vi "0MAIN.vi"() -> ()   [LabVIEW 2014]
uses:
  <vilib>/Instr/_visa.llb/VISA Configure Serial Port (Instr).vi
  <vilib>/Instr/_visa.llb/VISA Open Access Mode.ctl
panel:
  out "Пересчитано":bool=TRUE
  out "Метка получена 2":bool
  out "Время старта":string
  out "Ошибка файла":errorcluster
  out "Метка получена":bool
  out "Файл данных":refnum<file>
  out "Файл журнала":refnum<file>
  out "Номер метки":bool=TRUE
  out "error out 2":errorcluster
  in  "Управление":enum32{"Отладка", "График", "Настройки"}(tab)
  in  "Пересчитать в частоты":bool
  in  "Частота метки 2":bool
  in  "Записать данные":bool
  in  "Очистка буфера":bool
  in  "Чтение данных":bool
  in  "Установить":string
  in  "Отправка":bool
  out "Данные с МК":string
  out "Развертка X (В/ГГц)":dbl[](array[numeric])
  out "Сигнал Y (В)":dbl[](array[numeric])
  out "Метки (В, ГГц)":dbl[][](array[numeric])
  in  "Частота метки":bool
  in  "Выход":bool
  in  "Расчет графика":bool
  out "Индикатор КСВН":T1(graph)
  in  "Путь к файлу данных":path
  in  "Путь к логу":path
  in  "Логирование":bool
  out "Ошибка":T2
  in  "Порт":refnum<visa-resource-name>
  in  "Скорость передачи (9600)":u32=9600
  in  "Символ окончания (\\n)":u8=10 format="%.0x"
  in  "Режим доступа":T3 items=["VISA Defaults"=0, "Exclusive Lock"=1, "Load Configured Settings"=4]
  in  "Бит данных (8)":u8=8 format="%.0x"
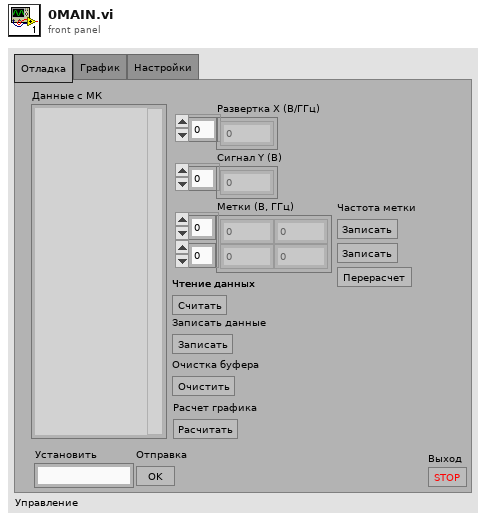
[diagram p1: front panel]
types:
  T1 = cluster{"Развертка X (В)":dbl[], "Сигнал Y (В)":dbl[]}
  T2 = cluster{"Статус":bool, "Код":i32, "Источник":string}
  T3 = typedef "VISA Open Access Mode.ctl" = u32
  T4 = enum16{"open", "replace", "create", "open or create", "replace or create", "replace or create with confirmation"}
  T5 = typedef "NI_Matrix.lvlib/RealMatrix.ctl" = dbl[][]
  T6 = cluster{"Развертка X (В/ГГц)":dbl[], "Сигнал Y (В)":dbl[]}
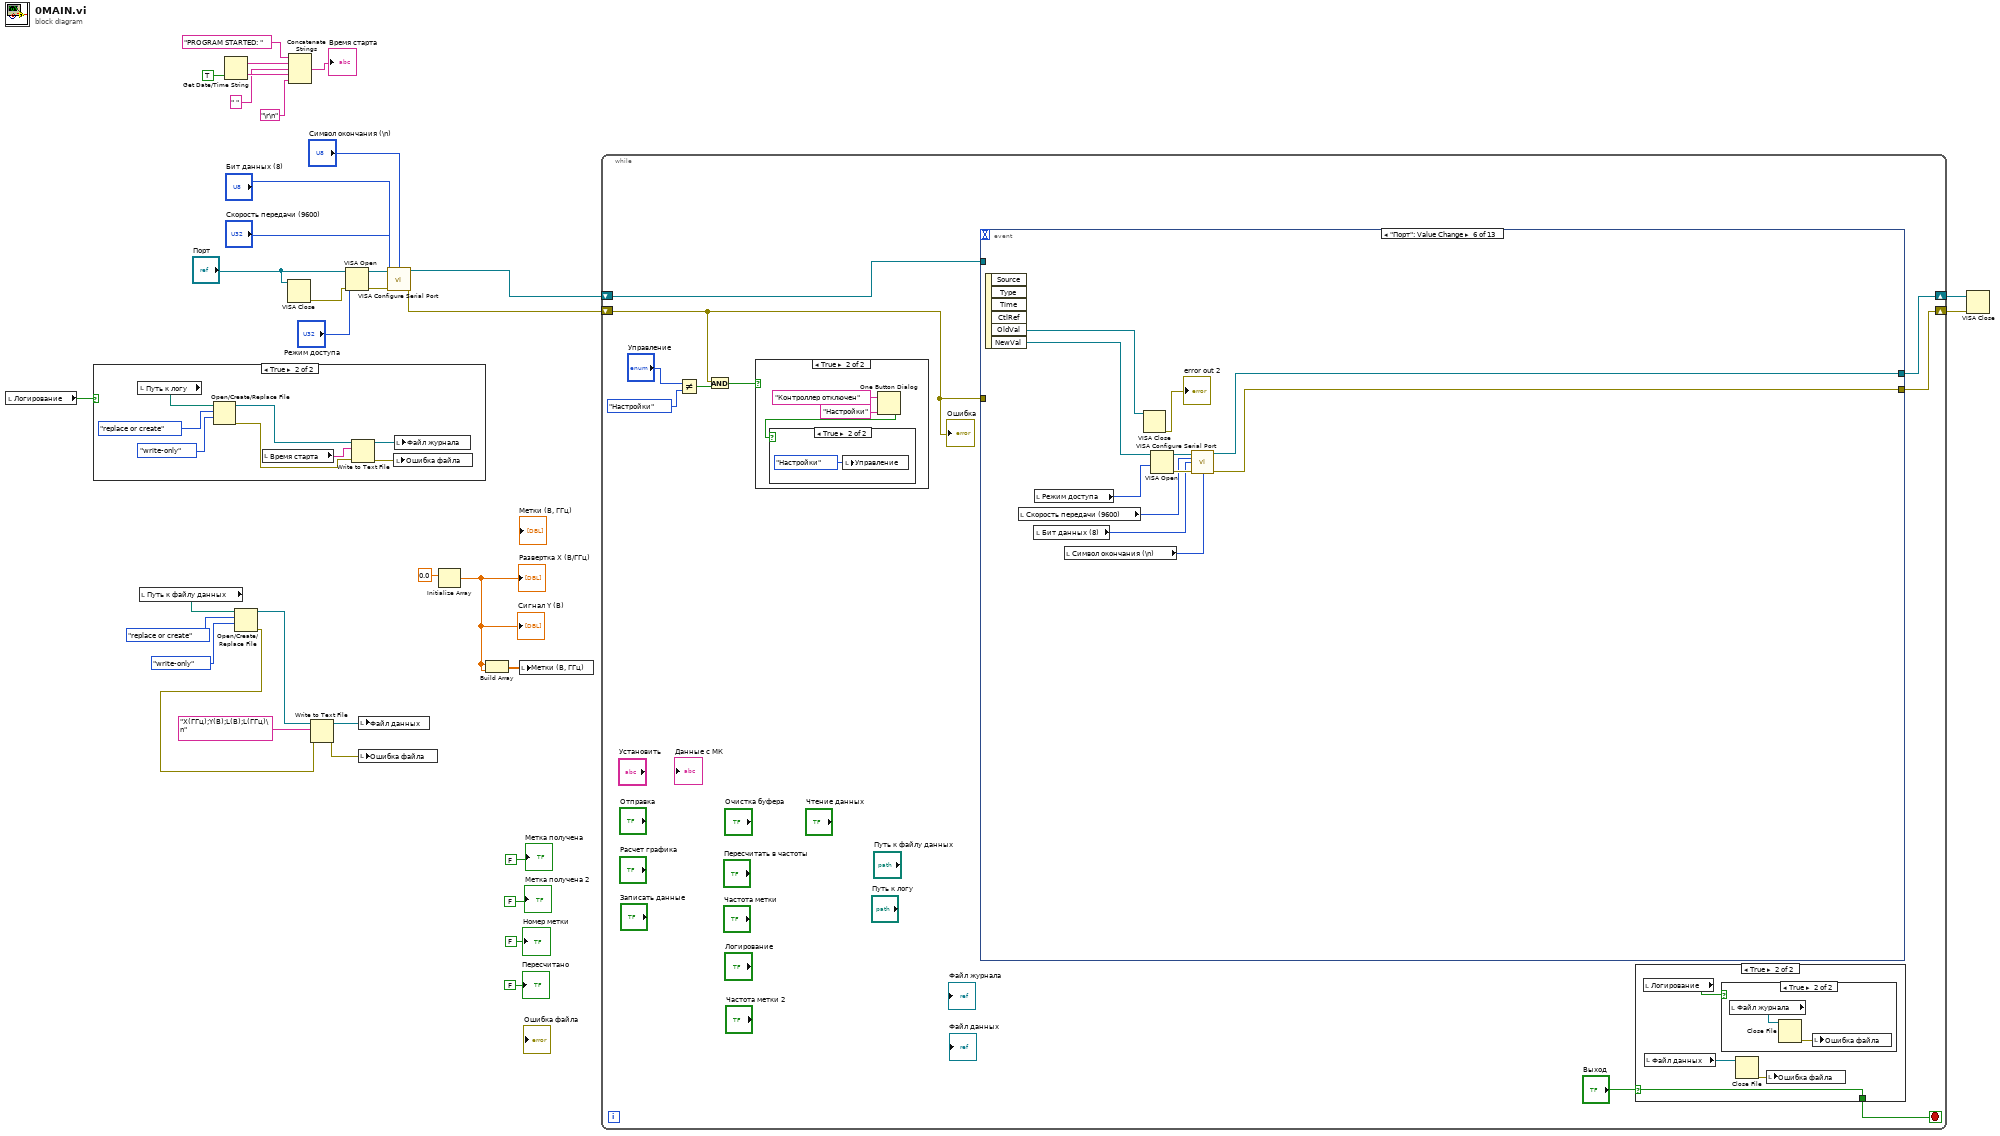
[diagram p0: block diagram]
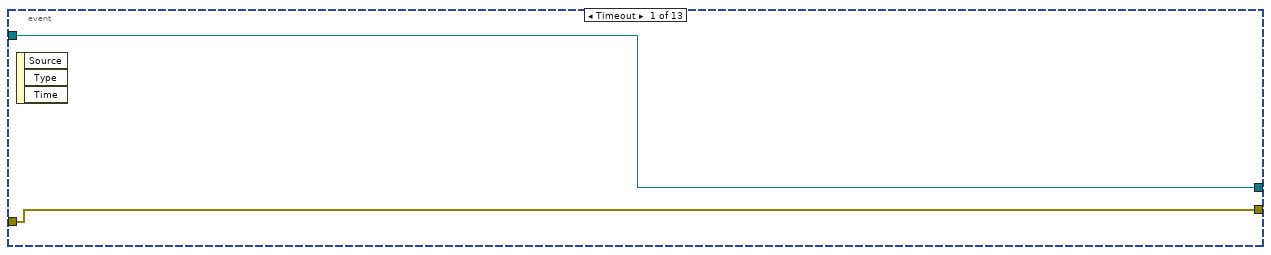
[diagram p7: hidden frame]
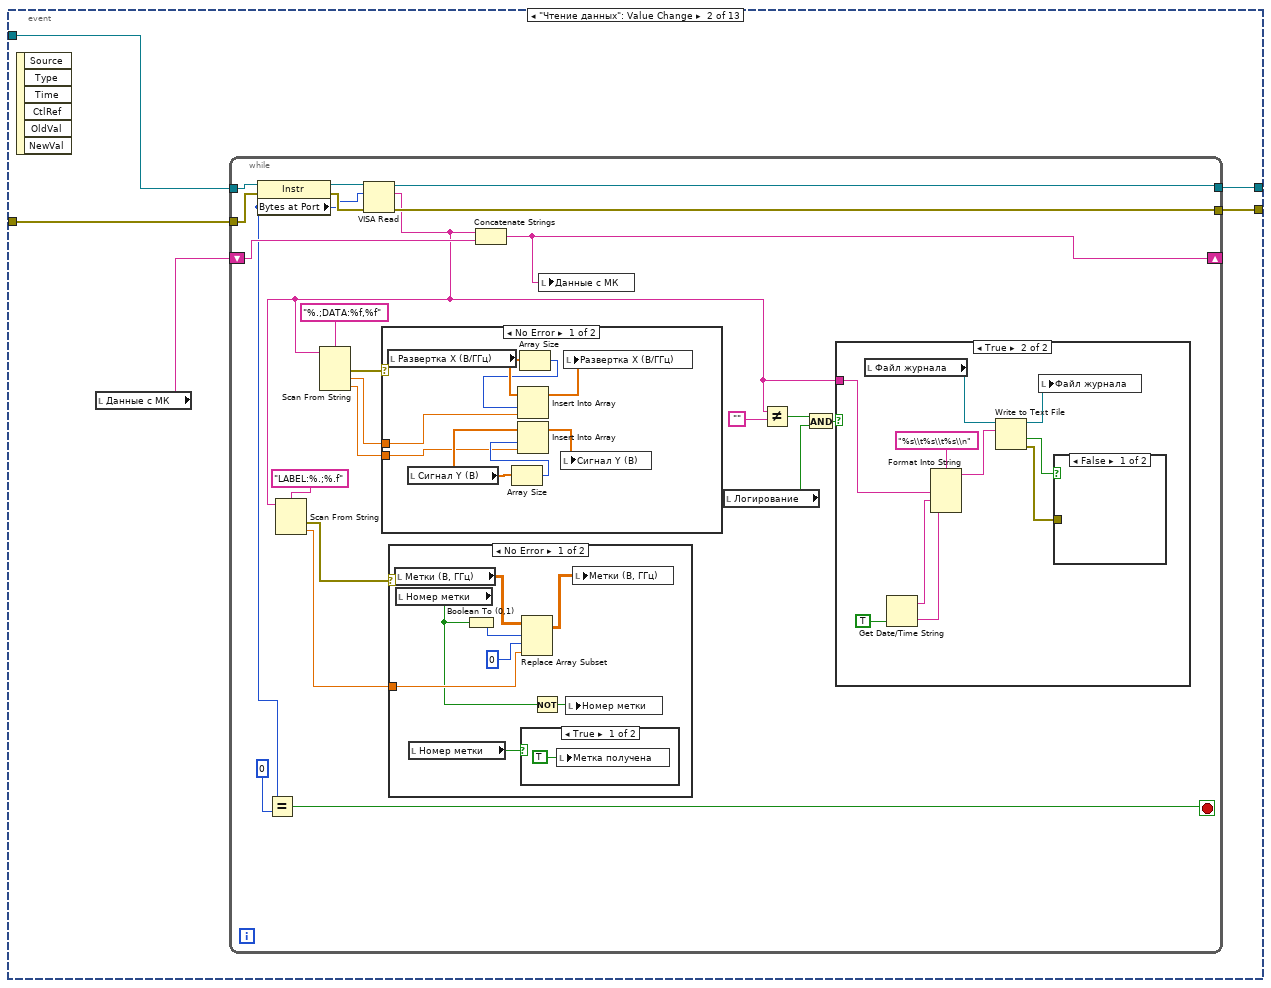
[diagram p8: hidden frame]
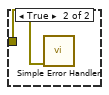
[diagram p10: hidden frame]
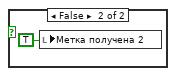
[diagram p11: hidden frame]
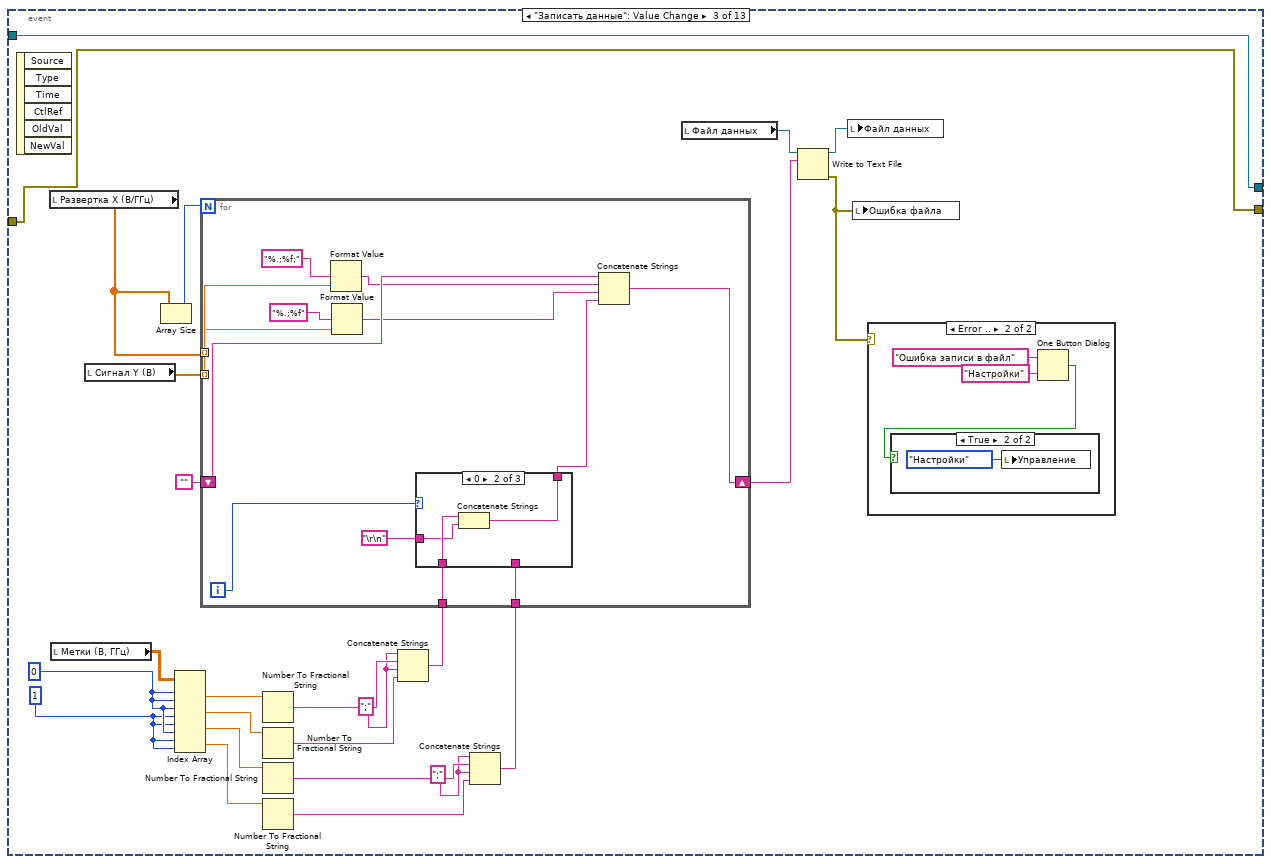
[diagram p14: hidden frame]
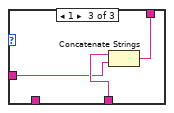
[diagram p18: hidden frame]
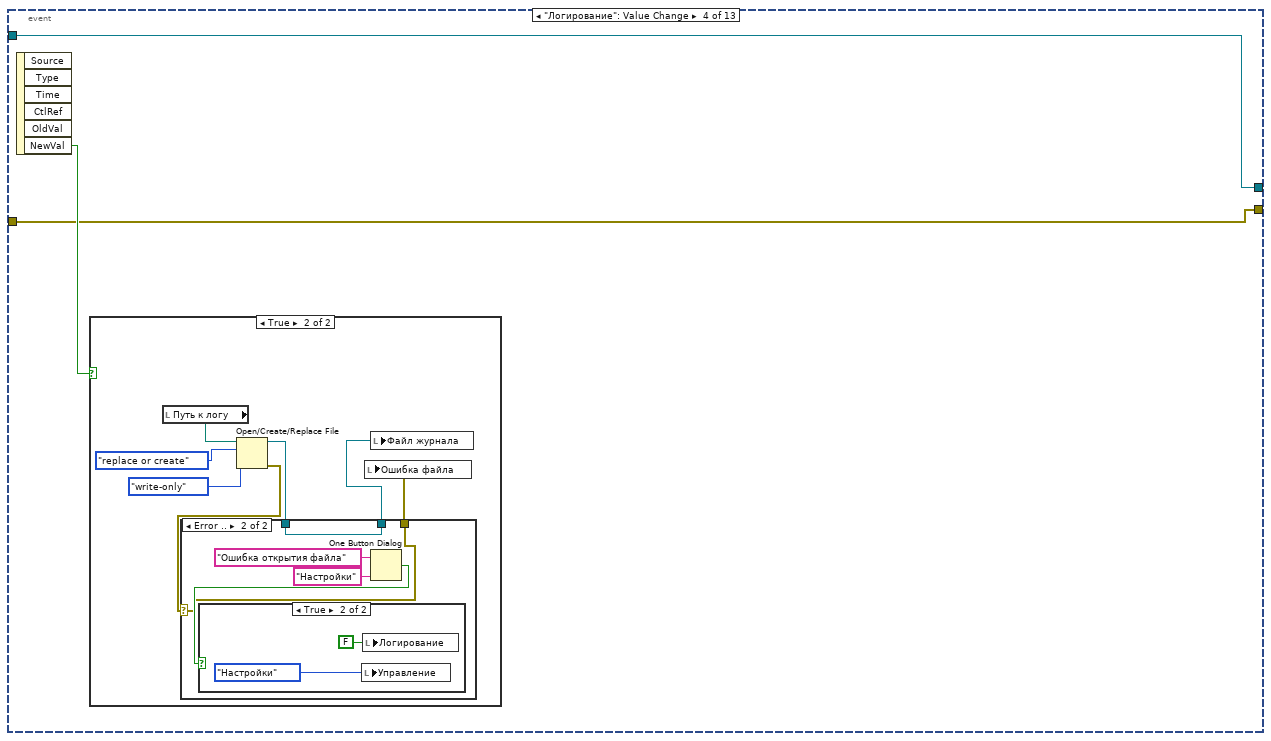
[diagram p19: hidden frame]
diagram:
  n1 = local read "Логирование"() -> (w13:bool)
  n2 = case shown="True" w13 {
    frame False {
    }
    frame True {
      n3 = local read "Путь к логу"() -> (w43:path)
      n4 = Open/Create/Replace File(file path (use dialog)=w43, operation (0:open)=T4."replace or create", access (0:read/write)=enum16{"read/write", "read-only", "write-only"}."write-only") -> (refnum out=w36:refnum<file>, error out=w37:errorcluster)  [unwired: 3 in, 1 out]
      n5 = local read "Время старта"() -> (w38:string)
      n6 = Write to Text File(file (use dialog)=w36, text=w38, error in=w37) -> (refnum out=w39:refnum<file>, error out=w40:errorcluster)  [unwired: 1 in, 1 out]
      n7 = local write "Ошибка файла"(w40) -> ()
      n8 = local write "Файл журнала"(w39) -> ()
    }
  }
  n9 = local read "Путь к файлу данных"() -> (w20:path)
  n10 = Get Date/Time String(want seconds? (F)=TRUE) -> (date string=w12:string, time string=w4:string)  [unwired: 2 in]
  n11 = Open/Create/Replace File(file path (use dialog)=w20, operation (0:open)=T4."replace or create", access (0:read/write)=enum16{"read/write", "read-only", "write-only"}."write-only") -> (refnum out=w6:refnum<file>, error out=w7:errorcluster)  [unwired: 3 in, 1 out]
  n12 = VISA Close(VISA resource name="Порт") -> (error out=w21:errorcluster)  [unwired: 1 in]
  n13 = Concatenate Strings("PROGRAM STARTED: " ("string"), w12, " ", w4, "\r\n" ("string")) -> (→"Время старта":string)
  n14 = Write to Text File(file (use dialog)=w6, text="X(ГГц);Y(В);L(В);L(ГГц)\n", error in=w7) -> (refnum out=w9:refnum<file>, error out=w10:errorcluster)  [unwired: 1 in, 1 out]
  n15 = VISA Open(access mode="Режим доступа", error in (no error)=w21, VISA resource name="Порт") -> (VISA resource name=w32:refnum<visa-resource-name>, error out=w31:errorcluster)  [unwired: 2 in]
  n16 = local write "Файл данных"(w9) -> ()
  n17 = local write "Ошибка файла"(w10) -> ()
  n18 = call-poly "VISA Configure Serial Port"("VISA resource name"=w32, "termination char\n(0xA = '\\n' = LF)"="Символ окончания (\\n)", "baud rate (9600)"="Скорость передачи (9600)", "data bits (8)"="Бит данных (8)", "error in (no error)"=w31) -> ("VISA resource name out"=w26:refnum<visa-resource-name>, "error out"=w28:errorcluster)  [unwired: 9 in]
  n19 = Initialize Array(0.0 ("element")) -> (w23:dbl[])  [unwired: 1 in]
  "Развертка X (В/ГГц)" <- w23
  "Сигнал Y (В)" <- w23
  n20 = Build Array(w23, w23) -> (w22:T5)
  n21 = local write "Метки (В, ГГц)"(w22) -> ()
  n22 = while {
    shift-right: [w45] -> w27
    shift-left: w28 -> [w49]
    shift-right: [w44] -> w25
    shift-left: w26 -> [w53]
    stop <- w46 stop-if-true
    n23 = Not Equal?(x="Управление", y=enum32{"Отладка", "График", "Настройки"}."Настройки" ("Tab Control")) -> (x != y?=w50:bool)
    n24 = And(x=w49, y=w50) -> (x .and. y?=w48:bool)
    n25 = case shown="True" w48 {
      frame False {
      }
      frame True {
        n26 = One Button Dialog(message="Контроллер отключен", button name ("OK")="Настройки") -> (true=w62:bool)
        n27 = case shown="True" w62 {
          frame False {
          }
          frame True {
            n28 = local write "Управление"(enum32{"Отладка", "График", "Настройки"}."Настройки" ("Tab Control")) -> ()
          }
        }
      }
    }
    n29 = event shown="[5] \"Порт\": Value Change" {
      selector: _ -> [_ _ _ _ _ _ _ _ _ _ _ _ _]
      dyn-events: _ -> [_ _ _ _ _ _ _ _ _ _ _ _ _]
      timeout: _ -> [_ _ _ _ _ _ _ _ _ _ _ _ _]
      tunnel: w49 -> [w66 w71 w124 w174 w195 _ w210 w219 w232 w237 w244 w269 w278]
      tunnel: [w66 w70 w124 w174 w195 w200 w210 w219 w232 w237 w244 w269 w277] -> w45
      tunnel: w53 -> [w65 w69 w125 w173 w196 _ w209 w220 w233 w238 w245 w270 w276]
      tunnel: [w65 w68 w125 w173 w196 w204 w209 w220 w233 w238 w245 w270 w275] -> w44
      event Timeout {
        n30 = event-data() -> ()  [unwired: 1 in, 3 out]
      }
      event "Чтение данных": Value Change {
        n31 = event-data() -> ()  [unwired: 1 in, 6 out]
        n32 = local read "Данные с МК"() -> (w67:string)
        n33 = while {
          tunnel: w69 -> [w89]
          tunnel: w71 -> [w88]
          tunnel: [w94] -> w68
          tunnel: [w93] -> w70
          shift-right: [w77] -> _
          shift-left: w67 -> [w92]
          stop <- w87 stop-if-true
          n34 = property class="Instr"(reference=w89, error in=w88) -> (reference out=w91:refnum<visa-resource-name>, error out=w90:errorcluster, "Bytes at Port"=w85:u32)
          n35 = Equal?(x=w85, y=u32 0 ("x")) -> (x = y?=w87:bool)
          n36 = VISA Read(VISA resource name=w91, byte count=w85, error in (no error)=w90) -> (VISA resource name out=w94:refnum<visa-resource-name>, read buffer=w73:string, error out=w93:errorcluster)  [unwired: 1 out]
          n37 = Scan From String(format string="LABEL:%.;%.f", input string=w73) -> (error out=w81:errorcluster, output 1=w80:dbl)  [unwired: 3 in, 2 out]
          n38 = Scan From String(format string="%.;DATA:%f,%f", input string=w73) -> (error out=w78:errorcluster, output 1=w84:dbl, output 2=w83:dbl)  [unwired: 4 in, 2 out]
          n39 = case shown="No Error" w78 {
            tunnel: w84 -> [w119 _]
            tunnel: w83 -> [w118 _]
            frame No Error {
              n40 = local read "Развертка X (В/ГГц)"() -> (w123:dbl[])
              n41 = local read "Сигнал Y (В)"() -> (w122:dbl[])
              n42 = Array Size(array=w122) -> (size(s)=w121:i32)
              n43 = Insert Into Array(array=w122, index=w121, new element=w118) -> (w116:dbl[])
              n44 = Array Size(array=w123) -> (size(s)=w120:i32)
              n45 = Insert Into Array(array=w123, index=w120, new element=w119) -> (w117:dbl[])
              n46 = local write "Сигнал Y (В)"(w116) -> ()
              n47 = local write "Развертка X (В/ГГц)"(w117) -> ()
            }
            frame Error {
            }
          }
          n48 = case shown="No Error" w81 {
            tunnel: w80 -> [w110 _]
            frame No Error {
              n49 = local read "Метки (В, ГГц)"() -> (w112:dbl[][])
              n50 = local read "Номер метки"() -> (w107:bool)
              n51 = local read "Номер метки"() -> (w106:bool)
              n52 = Boolean To (0,1)(Boolean=w107) -> (0, 1=w111:i16)
              n53 = case shown="True" w106 {
                frame True {
                  n54 = local write "Метка получена"(TRUE ("Метка получена")) -> ()
                }
                frame False {
                  n55 = local write "Метка получена 2"(TRUE ("Метка получена")) -> ()
                }
              }
              n56 = Replace Array Subset(array=w112, new element=w110, index (row)=w111, index (col)=0 ("disabled index (col)")) -> (w113:T5)
              n57 = Not(x=w107) -> (.not. x?=w108:bool)
              n58 = local write "Номер метки"(w108) -> ()
              n59 = local write "Метки (В, ГГц)"(w113) -> ()
            }
            frame Error {
            }
          }
          n60 = Concatenate Strings(w73, w92) -> (w77:string)
          n61 = local write "Данные с МК"(w77) -> ()
          n62 = local read "Логирование"() -> (w72:bool)
          n63 = Not Equal?(x=w73, y="") -> (x != y?=w75:bool)
          n64 = And(x=w75, y=w72) -> (x .and. y?=w76:bool)
          n65 = case shown="True" w76 {
            tunnel: w73 -> [_ w95]
            frame False {
            }
            frame True {
              n66 = local read "Файл журнала"() -> (w100:refnum<file>)
              n67 = Get Date/Time String(want seconds? (F)=TRUE) -> (date string=w99:string, time string=w98:string)  [unwired: 2 in]
              n68 = Format Into String(format string="%s\\t%s\\t%s\\n", w95, w99, w98) -> (resulting string=w96:string)  [unwired: 2 in, 1 out]
              n69 = Write to Text File(file (use dialog)=w100, text=w96) -> (refnum out=w101:refnum<file>, cancelled=w103:bool, error out=w102:errorcluster)  [unwired: 2 in]
              n70 = local write "Файл журнала"(w101) -> ()
              n71 = case shown="False" w103 {
                tunnel: w102 -> [_ w105]
                frame False {
                }
                frame True {
                  n72 = call <vilib>:"Simple Error Handler.vi"("error in (no error)"=w105) -> ()  [unwired: 4 in, 5 out]
                }
              }
            }
          }
        }
      }
      event "Записать данные": Value Change {
        w130 = ";"
        w131 = ";"
        w142 = 1
        w143 = 0
        n73 = event-data() -> ()  [unwired: 1 in, 6 out]
        n74 = local read "Развертка X (В/ГГц)"() -> (w146:dbl[])
        n75 = local read "Метки (В, ГГц)"() -> (w129:dbl[][])
        n76 = local read "Сигнал Y (В)"() -> (w147:dbl[])
        n77 = Array Size(array=w146) -> (size(s)=w148:i32)
        n78 = Index Array(array=w129, index (row) #1=w143, index (col) #1=w143, index (row) #2=w143, index (col) #2=w142, index (row) #3=w142, index (col) #3=w143, index (row) #4=w142, index (col) #4=w142) -> (element #1=w141:dbl, element #2=w140:dbl, element #3=w139:dbl, element #4=w138:dbl)
        n79 = Number To Fractional String(number=w141) -> (F-format string=w134:string)  [unwired: 3 in]
        n80 = Number To Fractional String(number=w140) -> (F-format string=w135:string)  [unwired: 3 in]
        n81 = Number To Fractional String(number=w139) -> (F-format string=w136:string)  [unwired: 3 in]
        n82 = Number To Fractional String(number=w138) -> (F-format string=w137:string)  [unwired: 3 in]
        n83 = Concatenate Strings(w130, w134, w130, w135) -> (w133:string)
        n84 = Concatenate Strings(w131, w136, w131, w137) -> (w132:string)
        n85 = for {
          N: w148 -> [_]
          tunnel: w147 -> [w164] mode=indexing
          tunnel: w146 -> [w165] mode=indexing
          shift-right: [w161] -> w128
          shift-left: "" -> [w156]
          tunnel: w133 -> [w159]
          tunnel: w132 -> [w158]
          i -> [w160]
          n86 = Format Value(format string="%.;%f;", value (0)=w165) -> (output string=w155:string)  [unwired: 1 in]
          n87 = Format Value(format string="%.;%f", value (0)=w164) -> (output string=w154:string)  [unwired: 1 in]
          n88 = case shown="0" w160 {
            tunnel: w159 -> [_ w169 _]
            tunnel: w158 -> [_ _ w172]
            tunnel: "\r\n" -> [w166 w168 w171]
            tunnel: [w166 w167 w170] -> w153
            frame Default {
            }
            frame 0 {
              n89 = Concatenate Strings(w169, w168) -> (w167:string)
            }
            frame 1 {
              n90 = Concatenate Strings(w172, w171) -> (w170:string)
            }
          }
          n91 = Concatenate Strings(w156, w155, w154, w153) -> (w161:string)
        }
        n92 = local read "Файл данных"() -> (w145:refnum<file>)
        n93 = Write to Text File(file (use dialog)=w145, text=w128) -> (refnum out=w144:refnum<file>, error out=w126:errorcluster)  [unwired: 2 in, 1 out]
        n94 = local write "Файл данных"(w144) -> ()
        n95 = local write "Ошибка файла"(w126) -> ()
        n96 = case shown="Error .." w126 {
          frame No Error {
          }
          frame Error {
            n97 = One Button Dialog(message="Ошибка записи в файл", button name ("OK")="Настройки") -> (true=w150:bool)
            n98 = case shown="True" w150 {
              frame False {
              }
              frame True {
                n99 = local write "Управление"(enum32{"Отладка", "График", "Настройки"}."Настройки" ("Управление")) -> ()
              }
            }
          }
        }
      }
      event "Логирование": Value Change {
        n100 = event-data() -> ("NewVal"=w175:bool)  [unwired: 1 in, 5 out]
        n101 = case shown="True" w175 {
          frame False {
          }
          frame True {
            n102 = local read "Путь к логу"() -> (w182:path)
            n103 = Open/Create/Replace File(file path (use dialog)=w182, operation (0:open)=T4."replace or create", access (0:read/write)=enum16{"read/write", "read-only", "write-only"}."write-only") -> (refnum out=w180:refnum<file>, error out=w181:errorcluster)  [unwired: 3 in, 1 out]
            n104 = case shown="Error .." w181 {
              selector: w181 -> [w186 w188]
              tunnel: w180 -> [w187 w189]
              tunnel: [w185 w188] -> w179
              tunnel: [w184 w189] -> w178
              frame No Error {
                n105 = local read "Время старта"() -> (w183:string)
                n106 = Write to Text File(file (use dialog)=w187, text=w183, error in=w186) -> (refnum out=w184:refnum<file>, error out=w185:errorcluster)  [unwired: 1 in, 1 out]
              }
              frame Error {
                n107 = One Button Dialog(message="Ошибка открытия файла", button name ("OK")="Настройки") -> (true=w191:bool)
                n108 = case shown="True" w191 {
                  frame False {
                  }
                  frame True {
                    n109 = local write "Управление"(enum32{"Отладка", "График", "Настройки"}."Настройки" ("Управление")) -> ()
                    n110 = local write "Логирование"(FALSE ("Логирование")) -> ()
                  }
                }
              }
            }
            n111 = local write "Ошибка файла"(w179) -> ()
            n112 = local write "Файл журнала"(w178) -> ()
          }
        }
      }
      event "Очистка буфера": Value Change {
        n113 = event-data() -> ()  [unwired: 1 in, 6 out]
        n114 = local write "Данные с МК"("") -> ()
      }
      event "Порт": Value Change {
        n115 = event-data() -> ("OldVal"=w199:refnum<visa-resource-name>, "NewVal"=w208:refnum<visa-resource-name>)  [unwired: 1 in, 4 out]
        n116 = local read "Скорость передачи (9600)"() -> (w203:u32)
        n117 = local read "Бит данных (8)"() -> (w202:u8)
        n118 = local read "Режим доступа"() -> (w207:T3)
        n119 = local read "Символ окончания (\\n)"() -> (w201:u8)
        n120 = VISA Close(VISA resource name=w199) -> (error out=→"error out 2":errorcluster)  [unwired: 1 in]
        n121 = VISA Open(access mode=w207, VISA resource name=w208) -> (VISA resource name=w206:refnum<visa-resource-name>, error out=w205:errorcluster)  [unwired: 3 in]
        n122 = call-poly "VISA Configure Serial Port"("VISA resource name"=w206, "termination char\n(0xA = '\\n' = LF)"=w201, "baud rate (9600)"=w203, "data bits (8)"=w202, "error in (no error)"=w205) -> ("VISA resource name out"=w204:refnum<visa-resource-name>, "error out"=w200:errorcluster)  [unwired: 9 in]
      }
      event "Частота метки": Value Change {
        n123 = event-data() -> ()  [unwired: 1 in, 6 out]
        n124 = local read "Метка получена"() -> (w211:bool)
        n125 = case shown="True" w211 {
          frame False {
          }
          frame True {
            n126 = local read "Установить"() -> (w217:string)
            n127 = local read "Метки (В, ГГц)"() -> (w213:dbl[][])
            n128 = Scan Value(string=w217, format string="%.;%f") -> (value=w218:dbl)  [unwired: 1 in, 1 out]
            n129 = Replace Array Subset(array=w213, new element=w218, index (row)=0 ("disabled index (row)"), index (col)=1 ("disabled index (col)")) -> (w214:T5)
            n130 = local write "Метки (В, ГГц)"(w214) -> ()
          }
        }
      }
      event "Частота метки 2": Value Change {
        n131 = event-data() -> ()  [unwired: 1 in, 6 out]
        n132 = local read "Метка получена 2"() -> (w221:bool)
        n133 = case shown="True" w221 {
          frame False {
          }
          frame True {
            n134 = local read "Установить"() -> (w227:string)
            n135 = local read "Метки (В, ГГц)"() -> (w223:dbl[][])
            n136 = Scan Value(string=w227, format string="%.;%f") -> (value=w228:dbl)  [unwired: 1 in, 1 out]
            n137 = Replace Array Subset(array=w223, new element=w228, index (row)=1 ("disabled index (row)"), index (col)=1 ("disabled index (col)")) -> (w224:T5)
            n138 = local write "Метки (В, ГГц)"(w224) -> ()
          }
        }
      }
      event "Расчет графика": Value Change {
        n139 = event-data() -> ()  [unwired: 1 in, 6 out]
        n140 = local read "Пересчитано"() -> (w229:bool)
        n141 = local read "Развертка X (В/ГГц)"() -> (w231:dbl[])
        n142 = local read "Сигнал Y (В)"() -> (w234:dbl[])
        n143 = case shown="False" w229 {
          frame False {
            n144 = property on="Индикатор КСВН" class="XYGraph (strict)"("XScale.NameLbl.Text"="Развертка Х, В" ("X Scale.Name Label.Text")) -> ()  [unwired: 2 in, 2 out]
          }
          frame True {
            n145 = property on="Индикатор КСВН" class="XYGraph (strict)"("XScale.NameLbl.Text"="Частота Х, ГГц" ("X Scale.Name Label.Text")) -> ()  [unwired: 2 in, 2 out]
          }
        }
        n146 = Bundle("Развертка X (В/ГГц)"=w231, "Сигнал Y (В)"=w234) -> (→"Индикатор КСВН":T6)  [unwired: 1 in]
      }
      event "Пересчитать в частоты": Value Change {
        n147 = event-data() -> ()  [unwired: 1 in, 6 out]
        n148 = local read "Развертка X (В/ГГц)"() -> (w242:dbl[])
        n149 = local read "Метки (В, ГГц)"() -> (w241:dbl[][])
        n150 = local write "Пересчитано"(TRUE ("Пересчитано")) -> ()
        n151 = Array Size(array=w242) -> (size(s)=w243:i32)
        n152 = formula code="float freq[1024];\nfloat umin,umax;\nfloat fmin, fmax;\numin = min(X[0],X[size-1]);\numax = max(X[0],X[size-1]);\nfmin = min(L[0][1], L[1][1]);\nfmax = max(L[0][1], L[1][1]);\nuInt8 i;\nfor (i = 0; i < size; i++) {\n     freq[i] = fmin+(X[i]-umin)/(umax-umin)*(fmax-fmin);\n};"("L"=w241, "X"=w242, "size"=w243) -> ("freq"=w240:dbl[])
        n153 = local write "Развертка X (В/ГГц)"(w240) -> ()
      }
      event "Путь к логу": Value Change {
        n154 = event-data() -> ("NewVal"=w246:path)  [unwired: 1 in, 5 out]
        n155 = local read "Логирование"() -> (w248:bool)
        n156 = case shown="True" w248 {
          selector: w248 -> [w257 w258]
          tunnel: [w257 w258] -> w247
          frame False {
          }
          frame True {
            n157 = local read "Файл журнала"() -> (w259:refnum<file>)
            n158 = Close File(refnum=w259) -> ()  [unwired: 1 in, 2 out]
          }
        }
        n159 = case shown="True" w247 {
          tunnel: w246 -> [_ w254]
          frame False {
          }
          frame True {
            n160 = local read "Время старта"() -> (w252:string)
            n161 = Open/Create/Replace File(file path (use dialog)=w254, operation (0:open)=T4."replace or create", access (0:read/write)=enum16{"read/write", "read-only", "write-only"}."write-only") -> (refnum out=w249:refnum<file>, error out=w251:errorcluster)  [unwired: 3 in, 1 out]
            n162 = Write to Text File(file (use dialog)=w249, text=w252, error in=w251) -> (refnum out=w250:refnum<file>, error out=w253:errorcluster)  [unwired: 1 in, 1 out]
            n163 = local write "Файл журнала"(w250) -> ()
            n164 = local write "Ошибка файла"(w253) -> ()
          }
        }
      }
      event "Путь к файлу данных": Value Change {
        n165 = event-data() -> ("NewVal"=w266:path)  [unwired: 1 in, 5 out]
        n166 = local read "Файл данных"() -> (w271:refnum<file>)
        n167 = Close File(refnum=w271) -> (error out=w260:errorcluster)  [unwired: 1 in, 1 out]
        n168 = local write "Ошибка файла"(w260) -> ()
        n169 = Open/Create/Replace File(file path (use dialog)=w266, operation (0:open)=T4."replace or create", access (0:read/write)=enum16{"read/write", "read-only", "write-only"}."write-only") -> (refnum out=w262:refnum<file>, error out=w264:errorcluster)  [unwired: 3 in, 1 out]
        n170 = Write to Text File(file (use dialog)=w262, text="X(ГГц);Y(В);L(В);L(ГГц)\n", error in=w264) -> (refnum out=w261:refnum<file>, error out=w263:errorcluster)  [unwired: 1 in, 1 out]
        n171 = local write "Файл данных"(w261) -> ()
        n172 = local write "Ошибка файла"(w263) -> ()
      }
      event "Отправка": Value Change {
        n173 = event-data() -> ()  [unwired: 1 in, 6 out]
        n174 = local read "Установить"() -> (w272:string)
        n175 = Equal?(x=w272, y="02") -> (x = y?=w273:bool)
        n176 = VISA Write(VISA resource name=w276, write buffer=w272, error in (no error)=w278) -> (VISA resource name out=w275:refnum<visa-resource-name>, error out=w277:errorcluster)  [unwired: 1 out]
        n177 = case shown="True" w273 {
          frame False {
          }
          frame True {
            n178 = Initialize Array(0.0 ("element")) -> (w280:dbl[])  [unwired: 1 in]
            n179 = local write "Развертка X (В/ГГц)"(w280) -> ()
            n180 = local write "Пересчитано"(FALSE ("Пересчитано")) -> ()
            n181 = local write "Сигнал Y (В)"(w280) -> ()
          }
        }
      }
    }
    n182 = case shown="True" "Выход" {
      selector: "Выход" -> [w54 w56]
      tunnel: [w54 w56] -> w46
      frame False {
      }
      frame True {
        n183 = local read "Логирование"() -> (w58:bool)
        n184 = local read "Файл данных"() -> (w57:refnum<file>)
        n185 = case shown="True" w58 {
          frame False {
          }
          frame True {
            n186 = local read "Файл журнала"() -> (w60:refnum<file>)
            n187 = Close File(refnum=w60) -> (error out=w59:errorcluster)  [unwired: 1 in, 1 out]
            n188 = local write "Ошибка файла"(w59) -> ()
          }
        }
        n189 = Close File(refnum=w57) -> (error out=w55:errorcluster)  [unwired: 1 in, 1 out]
        n190 = local write "Ошибка файла"(w55) -> ()
      }
    }
    "Ошибка" <- w49
  }
  n191 = VISA Close(VISA resource name=w25, error in (no error)=w27) -> ()  [unwired: 1 out]
  "Номер метки" <- FALSE ("Номер метки")
  "Метка получена" <- FALSE ("Частоты определены")
  "Метка получена 2" <- FALSE ("Частоты определены")
  "Пересчитано" <- FALSE ("Номер метки")
